vi "Notify FGV.vi"(7 "Actions":T1(ring)=enum."Send", 8 "error in":errorcluster, 10 "notification":variant) -> (0 "error out":errorcluster, 3 "notifier out":refnum<notifier>)   [LabVIEW 2019, in "Sequencer Handshake.lvlib"]
doc: "Notifier FGV with the following functions:\n\n-Obtain: Create reference for the notifier.\n-Send: Send notification with the FGV reference.\n-Get Notifier: Get the notifier reference (No operation is performed).\n-Release: Release notifier reference.\n\nNote: The current notifier reference can be obtained with every action if required, but the get notifier action was designed just for this purpose.\n\n-----\nJuan Navarro\nLab it Studio"
uses:
  Sequencer Handshake.lvlib
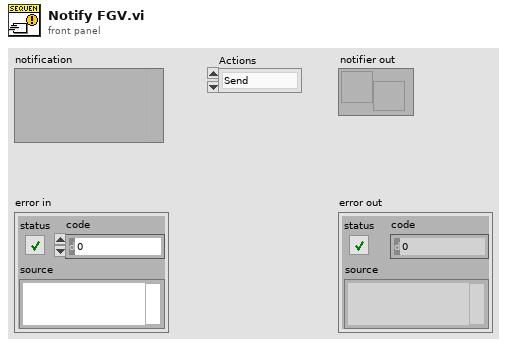
[diagram p1: front panel]
types:
  T1 = enum16{"Obtain", "Send", "Get Notifier", "Release"}
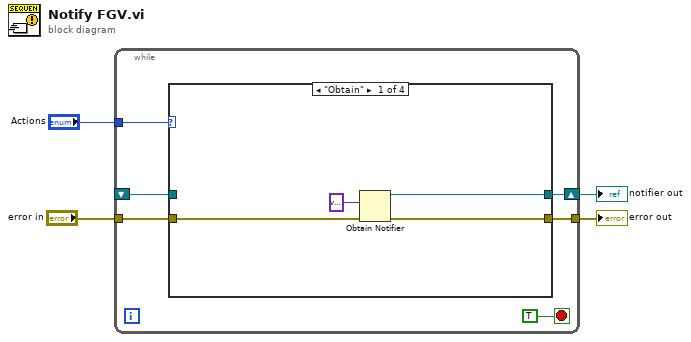
[diagram p0: block diagram]
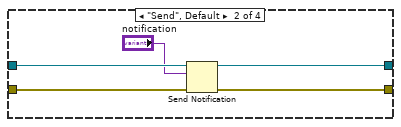
[diagram p2: hidden frame]
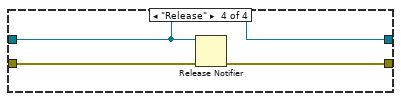
[diagram p4: hidden frame]
diagram:
  n1 = while {
    tunnel: "Actions" -> [w10]
    tunnel: [w9] -> w2
    shift-right: [w8] -> w1
    shift-left: _ -> [w6]
    tunnel: "error in" -> [w7]
    stop <- TRUE stop-if-true
    n2 = case shown="\"Obtain\"" w10 {
      tunnel: w7 -> [w13 w19 w20 w24]
      tunnel: [w12 w18 w20 w23] -> w9
      tunnel: [w11 w16 w21 w22] -> w8
      tunnel: w6 -> [_ w17 w21 w22]
      frame "Obtain" {
        n3 = Obtain Notifier(notification data type=variant ("element data type"), error in (no error)=w13) -> (notifier out=w11:refnum<notifier>, error out=w12:errorcluster)  [unwired: 2 in, 1 out]
      }
      frame "Send", Default {
        n4 = Send Notification(notification="notification", notifier=w17, error in (no error)=w19) -> (notifier out=w16:refnum<notifier>, error out=w18:errorcluster)
      }
      frame "Get Notifier" {
      }
      frame "Release" {
        n5 = Release Notifier(notifier=w22, error in (no error)=w24) -> (error out=w23:errorcluster)  [unwired: 1 in, 2 out]
      }
    }
  }
  "error out" <- w2
  "notifier out" <- w1
